vi "MassCompile--function.vi"(8 "error in":errorcluster, 9 "Number of VIs to Cache":u32=100, 10 "Mass Compile Log File":path, 11 "Directory to Compile":path) -> (0 "error out":errorcluster, 2 "log text":string)   [LabVIEW 2020, in "CICD.lvlib"]
doc: "Invoke Mass Compile operation and spit out results in text format."
uses:
  CICD.lvlib
  <vilib>/Utility/error.llb/Error Cluster From Error Code.vi
  <vilib>/ErrorRing/Error Ring.xnode
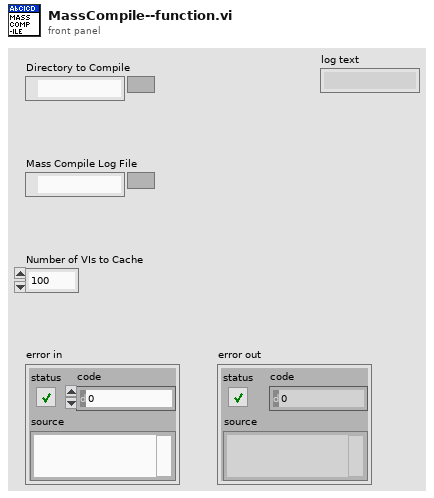
[diagram p1: front panel]
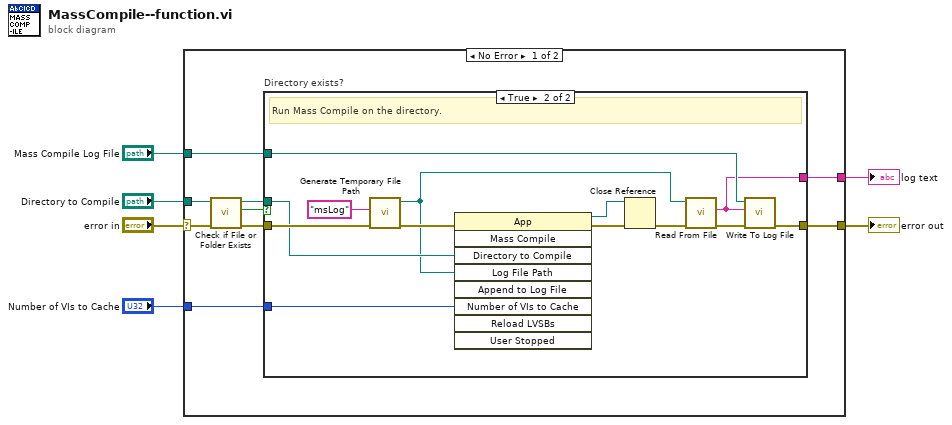
[diagram p0: block diagram]
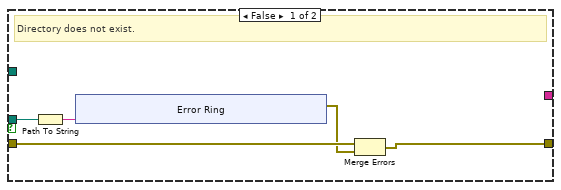
[diagram p2: hidden frame]
diagram:
  n1 = case shown="No Error" "error in" {
    selector: "error in" -> [w13 w41]
    tunnel: [w15 w41] -> w6
    tunnel: "Number of VIs to Cache" -> [w12 _]
    tunnel: "Directory to Compile" -> [w10 _]
    tunnel: "Mass Compile Log File" -> [w8 _]
    tunnel: [w7 _] -> w1
    frame No Error {
      n2 = call <vilib>:"Check if File or Folder Exists.vi"("error in (no error)"=w13, "path"=w10) -> ("error out"=w14:errorcluster, "file or folder exists?"=w11:bool, "dup path"=w9:path)  [unwired: 7 in]
      n3 = case "Directory exists?" shown="True" w11 {
        tunnel: [w19 w35] -> w15
        tunnel: w9 -> [w17 w32]
        tunnel: w12 -> [_ w31]
        tunnel: w14 -> [w20 w38]
        tunnel: w8 -> [_ w29]
        tunnel: [_ w28] -> w7
        frame False {
          # "Directory does not exist."
          n4 = Path To String(path=w17) -> (string=w16:string)
          n5 = xnode "Error Ring"("parameter 0"=w16) -> ("error out"=w18:errorcluster)
          n6 = Merge Errors(w20, w18) -> (w19:errorcluster)
        }
        frame True {
          # "Run Mass Compile on the directory."
          n7 = call <vilib>:"Generate Temporary File Path.vi"("error in (no error)"=w38, "Temporary File Extension (tmp)"="msLog") -> ("error out"=w40:errorcluster, "Unique Temporary File Path"=w30:path)  [unwired: 8 in]
          n8 = invoke class="App" method="Mass Compile"(error in=w40, "Directory to Compile"=w32, "Log File Path"=w30, "Number of VIs to Cache"=w31) -> (reference out=w33:refnum<vi>, error out=w39:errorcluster)  [unwired: 5 in, 7 out]
          n9 = Close Reference(reference=w33, error in (no error)=w39) -> (error out=w37:errorcluster)
          n10 = call "Read From File.vi"("error in"=w37, "file path"=w30) -> ("error out"=w36:errorcluster, "text"=w28:string)  [unwired: 8 in]
          n11 = call "Write To Log File.vi"("error in"=w36, "log text"=w28, "file path"=w29) -> ("error out"=w35:errorcluster)  [unwired: 8 in]
        }
      }
    }
    frame Error {
    }
  }
  "error out" <- w6
  "log text" <- w1
